vi "main.vi"() -> ()   [LabVIEW 2023]
panel:
  in  "Direction":string
  in  "Line Number":string
  in  "Stop ID":string
  out "ETA to\nNext Tram\n(Minutes)":dbl
  in  "Get Button":bool
  # "Inputs"
  # "Results"
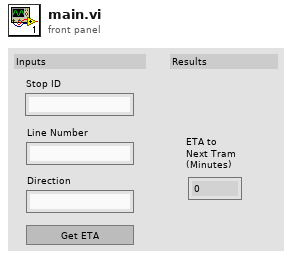
[diagram p1: front panel]
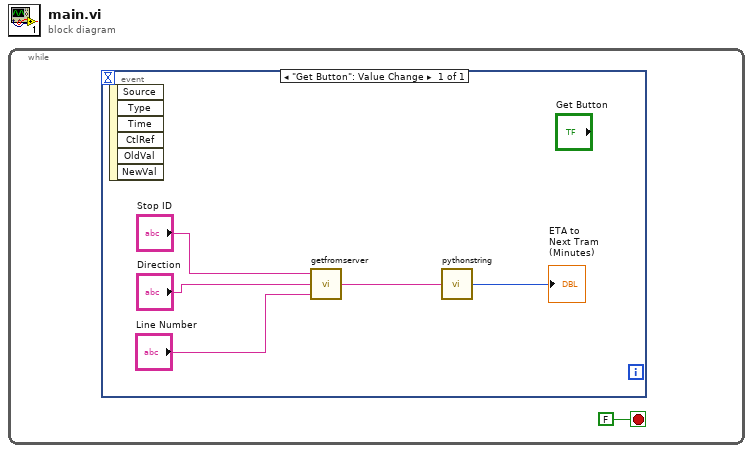
[diagram p0: block diagram]
diagram:
  n1 = while {
    stop <- FALSE stop-if-true
    n2 = event shown="[0] \"Get Button\": Value Change" {
      selector: _ -> [_]
      dyn-events: _ -> [_]
      timeout: _ -> [_]
      event "Get Button": Value Change {
        n3 = event-data() -> ()  [unwired: 1 in, 6 out]
        n4 = call "getfromserver.vi"("Line Number"="Line Number", "Direction"="Direction", "Stop ID"="Stop ID") -> ("Result Body"=w6:string)
        n5 = call "pythonstring.vi"("Result Body"=w6) -> ("ETA"=→"ETA to\nNext Tram\n(Minutes)":i32)
      }
    }
  }
